vi "Costo Update.vi"(8 "error in (no error)":errorcluster, 10 "Costo":dbl, 11 "UI in":refnum<class "UI.lvclass">) -> (0 "error out":errorcluster, 3 "UI out":refnum<class "UI.lvclass">)   [LabVIEW 2021, in "UI.lvlib" / "UI.lvclass"]
uses:
  UI.lvclass
  UI.lvclass/UI.ctl
  Monedas Messages/Actualizacion Credito Msg/Actualizacion Credito Msg.lvclass/Actualizacion Credito Msg.ctl
  <vilib>/ActorFramework/Message Enqueuer/Message Enqueuer.lvclass/Message Enqueuer.ctl
  Productos Messages/Actualizacion Costos Msg/Actualizacion Costos Msg.lvclass/Actualizacion Costos Msg.ctl
  Mensajes Messages/Mensaje arrive Msg/Mensaje arrive Msg.lvclass/Mensaje arrive Msg.ctl
  <vilib>/ActorFramework/Message Enqueuer/Enqueue.vi
  Monedas Messages/Actualizacion Credito Msg/Actualizacion Credito Msg.lvclass
  C:/Program Files (x86)/National Instruments/LabVIEW 2021/vi.lib/ActorFramework/Message/Message.lvclass
  Productos Messages/Actualizacion Costos Msg/Actualizacion Costos Msg.lvclass
  Mensajes Messages/Mensaje arrive Msg/Mensaje arrive Msg.lvclass
  <vilib>/ActorFramework/Message Priority Queue/Priority Enqueue.vi
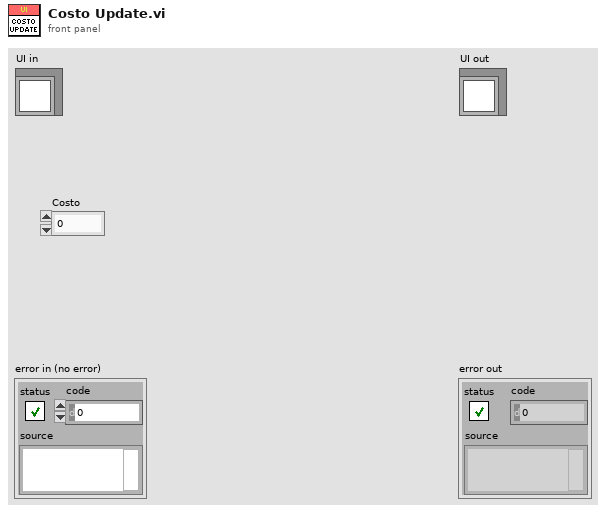
[diagram p1: front panel]
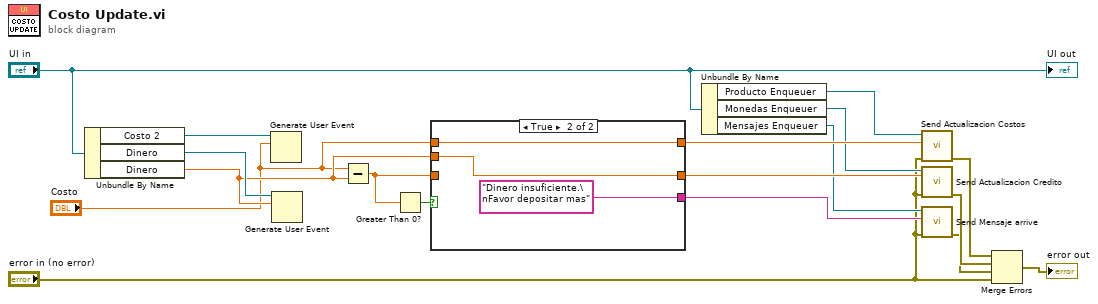
[diagram p0: block diagram]
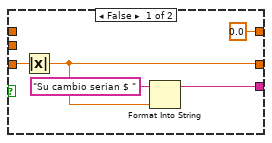
[diagram p2: hidden frame]
diagram:
  n1 = Unbundle By Name("UI in") -> ("Costo 2"=w18:refnum<user-event>, "Dinero"=w17:refnum<user-event>, "Dinero"=w14:dbl)
  n2 = Generate User Event(user event=w18, event data cluster="Costo") -> ()  [unwired: 2 in, 2 out]
  n3 = Generate User Event(user event=w17, event data cluster=w14) -> ()  [unwired: 2 in, 2 out]
  n4 = Subtract(x="Costo", y=w14) -> (x-y=w15:dbl)
  n5 = Greater Than 0?(x=w15) -> (x > 0?=w16:bool)
  n6 = case shown="True" w16 {
    tunnel: w15 -> [w21 _]
    tunnel: [w20 w26] -> w11
    tunnel: w14 -> [_ w26]
    tunnel: "Costo" -> [_ w25]
    tunnel: [0.0 ("Costo") w25] -> w12
    tunnel: [w19 "Dinero insuficiente.\nFavor depositar mas" ("message")] -> w5
    frame False {
      n7 = Absolute Value(x=w21) -> (abs(x)=w20:dbl)
      n8 = Format Into String(initial string="Su cambio serian $ ", w20) -> (resulting string=w19:string)  [unwired: 2 in, 1 out]
    }
    frame True {
    }
  }
  n9 = Unbundle By Name("UI in") -> ("Producto Enqueuer"=w8:refnum<class "Message Enqueuer.lvclass">, "Monedas Enqueuer"=w7:refnum<class "Message Enqueuer.lvclass">, "Mensajes Enqueuer"=w6:refnum<class "Message Enqueuer.lvclass">)
  n10 = call "Send Actualizacion Costos.vi"("error in (no error)"="error in (no error)", "Costo"=w12, "Message Enqueuer"=w8) -> ("error out"=w4:errorcluster)  [unwired: 7 in, 1 out]
  n11 = call "Send Actualizacion Credito.vi"("error in (no error)"="error in (no error)", "Credito"=w11, "Message Enqueuer"=w7) -> ("error out"=w3:errorcluster)  [unwired: 7 in, 1 out]
  n12 = call "Send Mensaje arrive.vi"("error in (no error)"="error in (no error)", "Palabra entrada"=w5, "Message Enqueuer"=w6) -> ("error out"=w2:errorcluster)  [unwired: 7 in, 1 out]
  n13 = Merge Errors(w4, w3, w2, "error in (no error)") -> (→"error out":errorcluster)
  "UI out" <- "UI in"
